vi "selectDevice.vi"(8 "error in (no error)":errorcluster, 9 "Custom Button 1":refnum<vi>, 10 "Custom Button 2":refnum<vi>, 11 "Daten in":T4={"Report.lvclass"=refnum, "Norm"="", "last State"=enum."Initialize", "Norm ID"=0, "EMTestCWS500N.lvclass"=refnum, "CEG4500.lvclass"=refnum, "Tektronix RSA5106A.lvclass"=refnum, "erfolgreich"=FALSE, "Device Enum"=enum."emTestCWS500N", "Test Enum"=enum."HF-Felder", "debug"=FALSE, "tab"=enum."Hauptmenü", "ESD Pistol.lvclass"=refnum, "SubPnl Refnum"=refnum, "TabCtl Refnum"=refnum, "ButtonsEinblenden?"=FALSE, "VKey"=enum."ASCII", "last Test"=refnum, "Class 4.lvclass"=refnum}) -> (0 "error out":errorcluster, 1 "DeviceInterface out":refnum<class "DeviceInterface.lvclass">, 2 "Burst.lvclass":refnum<class "TestInterface.lvclass">, 3 "Daten out":T4={"Report.lvclass"=refnum, "Norm"="", "last State"=enum."Initialize", "Norm ID"=0, "EMTestCWS500N.lvclass"=refnum, "CEG4500.lvclass"=refnum, "Tektronix RSA5106A.lvclass"=refnum, "erfolgreich"=FALSE, "Device Enum"=enum."emTestCWS500N", "Test Enum"=enum."HF-Felder", "debug"=FALSE, "tab"=enum."Hauptmenü", "ESD Pistol.lvclass"=refnum, "SubPnl Refnum"=refnum, "TabCtl Refnum"=refnum, "ButtonsEinblenden?"=FALSE, "VKey"=enum."ASCII", "last Test"=refnum, "Class 4.lvclass"=refnum}, 4 "Test Enum":T1, 5 "VISA resource name":refnum<visa-resource-name>, 6 "Device Enum":T2)   [LabVIEW 2013, in "EMV-Test.lvlib"]
uses:
  EMV-Test.lvlib
  classes/Devices/DeviceInterface/DeviceInterface.lvclass
  classes/Tests/Stoeraussendung/Stoeraussendung.lvclass
  classes/Tests/TestInterface/TestInterface.lvclass
  classes/Tests/Burst/Burst.lvclass
  classes/Tests/ESD/ESD.lvclass
  classes/Tests/Surge/Surge.lvclass
  classes/Tests/Spannungseinbruch/Spannungseinbruch.lvclass
  classes/Tests/HF-Felder/HF-Felder.lvclass
  Main/controls/TestStates.ctl
  classes/Tests/TestTest/TestTest.lvclass
  classes/Datastructure/Report/Report.lvclass
  Main/controls/State.ctl
  classes/Devices/emTestCWS500N/EMTestCWS500N.lvclass
  classes/Devices/CEG4500/CEG4500.lvclass
  classes/Devices/Tektronix RSA5106A/Tektronix RSA5106A.lvclass
  classes/Devices/DeviceInterface/Devices.ctl
  classes/Tests/TestInterface/Tests.ctl
  Main/controls/Data.ctl
  vis/Tabs.ctl
  vis/ESD Pistol.lvclass
  <vilib>/event_ctls.llb/eventvkey.ctl
  classes/Datastructure/Test/Test.lvclass
  classes/Devices/Class4/Class 4.lvclass
panel:
  out "Enum":T3
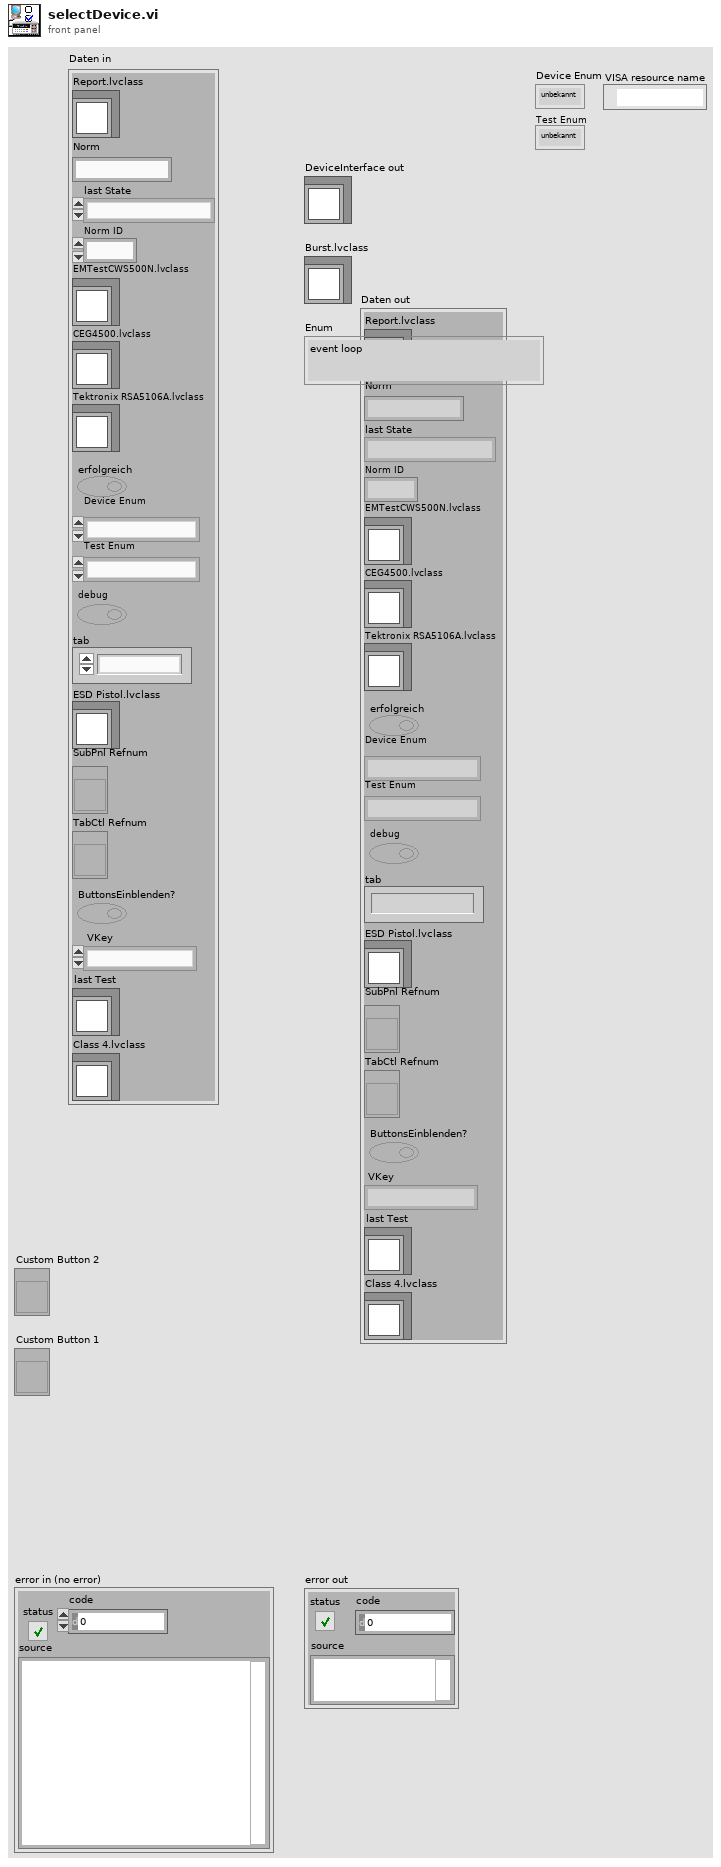
[diagram p1: front panel]
types:
  T1 = typedef "Tests.ctl" = enum16{"unbekannt", "Störaussendung", "Burst", "ESD", "Surge", "Spannungseinbruch", "HF-Felder"}
  T2 = typedef "Devices.ctl" = enum16{"unbekannt", "ESD Pistol", "Tektronix RSA5106A", "emTestCWS500N", "CEG-4500"}
  T3 = typedef "EMV-Test.lvlib/TestStates.ctl" = enum16{"event loop", "save Test", "Custom Action 1", "Custom Action 2", "pause", "vorgefertigter Test", "manueller Test", "respond to response", "error", "init", "start Test", "evaluate line", "wait for Response", "wait", "catch error", "close Connection", "end"}
  T4 = typedef "Data.ctl" = cluster{"Report.lvclass":refnum<class "Report.lvclass">, "Norm":string, "last State":T5, "Norm ID":i32, "EMTestCWS500N.lvclass":refnum<class "EMTestCWS500N.lvclass">, "CEG4500.lvclass":refnum<class "CEG4500.lvclass">, "Tektronix RSA5106A.lvclass":refnum<class "Tektronix RSA5106A.lvclass">, "erfolgreich":bool, "Device Enum":T2, "Test Enum":T1, "debug":bool, "tab":T6, "ESD Pistol.lvclass":refnum<class "ESD Pistol.lvclass">, "SubPnl Refnum":refnum<vi>, "TabCtl Refnum":refnum<vi>, "ButtonsEinblenden?":bool, "VKey":T7, "last Test":refnum<class "Test.lvclass">, "Class 4.lvclass":refnum<class "Class 4.lvclass">}
  T5 = typedef "State.ctl" = enum16{"create Pdf", "edit Report", "load Report", "save Report", "do Test", "CDN Kalibrierung", "enter Report Parameters", "new Test", "Protokoll", "read Tree", "update Tree", "Fehler", "Initialize", "Wait for Event", "Exit"}
  T6 = typedef "Tabs.ctl" = enum32{"Hauptmenü", "Prüfbericht", "Einstellungen"}
  T7 = typedef "eventvkey.ctl" = enum16{"ASCII", "Enter", "Return", "Shift", "Ctrl", "Alt", "Cmd", "Opt", "Caps", "NumLock", "Clear", "Break", "Up", "Down", "Left", "Right", "Insert", "Delete", "Home", "End", "PageUp", "PageDown", "Escape", "Help", "Pause", "ScrollLock", "F1", "F2", "F3", "F4", "F5", "F6", "F7", "F8", "F9", "F10", "F11", "F12", "F13", "F14", "F15", "F16", "F17", "F18", "F19", "F20", "F21", "F22", "F23", "F24", "Play", "VolumeUp", "VolumeDown", "Mute", "Two Byte Char"}
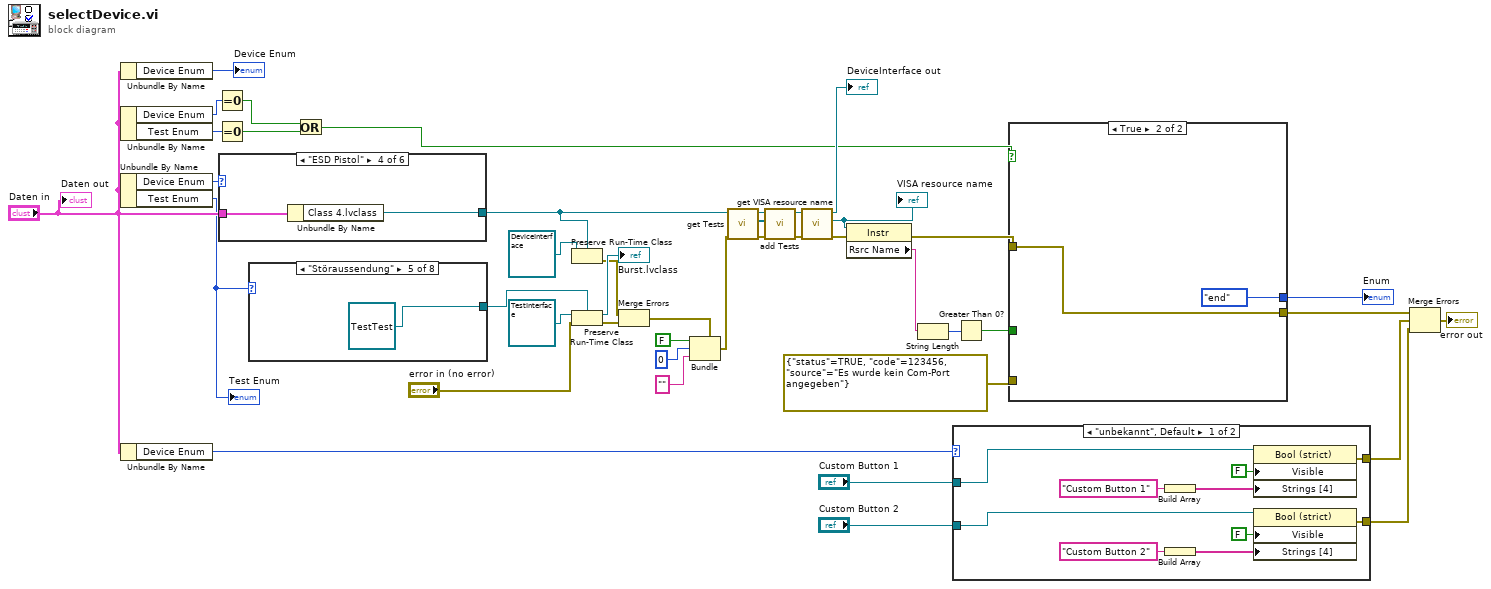
[diagram p0: block diagram]
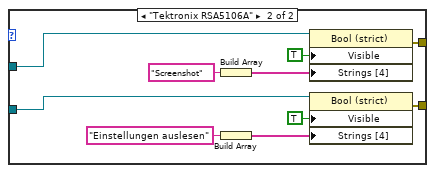
[diagram p2: hidden frame]
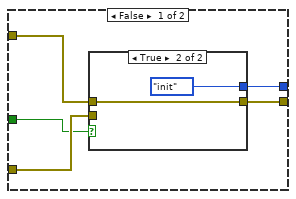
[diagram p3: hidden frame]
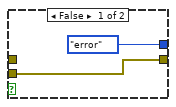
[diagram p4: hidden frame]
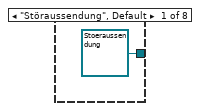
[diagram p5: hidden frame]
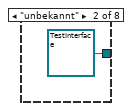
[diagram p6: hidden frame]
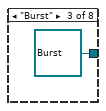
[diagram p7: hidden frame]
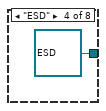
[diagram p8: hidden frame]
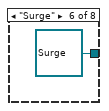
[diagram p9: hidden frame]
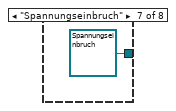
[diagram p10: hidden frame]
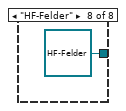
[diagram p11: hidden frame]
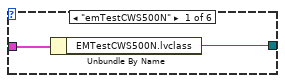
[diagram p12: hidden frame]
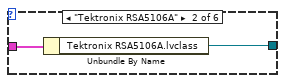
[diagram p13: hidden frame]
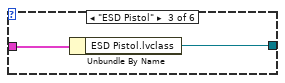
[diagram p14: hidden frame]
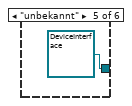
[diagram p15: hidden frame]
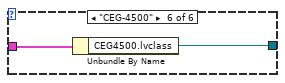
[diagram p16: hidden frame]
diagram:
  n1 = Unbundle By Name("Daten in") -> ("Device Enum"=→"Device Enum":T2)
  n2 = Unbundle By Name("Daten in") -> ("Device Enum"=w18:T2, "Test Enum"=w21:T1)
  n3 = Unbundle By Name("Daten in") -> ("Device Enum"=w28:T2, "Test Enum"=w29:T1)
  "Test Enum" <- w29
  n4 = Unbundle By Name("Daten in") -> ("Device Enum"=w33:T2)
  n5 = Equal To 0?(x=w18) -> (x = 0?=w19:bool)
  n6 = Equal To 0?(x=w21) -> (x = 0?=w20:bool)
  n7 = case shown="\"ESD Pistol\"" w28 {
    tunnel: [w44 w46 w48 w50 refnum<class "DeviceInterface.lvclass"> refnum ("Tektronix RSA5106A.lvclass") w53] -> w30
    tunnel: "Daten in" -> [w45 w47 w49 w51 _ w54]
    frame "emTestCWS500N" {
      n8 = Unbundle By Name(w45) -> ("EMTestCWS500N.lvclass"=w44:refnum<class "EMTestCWS500N.lvclass">)
    }
    frame "Tektronix RSA5106A" {
      n9 = Unbundle By Name(w47) -> ("Tektronix RSA5106A.lvclass"=w46:refnum<class "Tektronix RSA5106A.lvclass">)
    }
    frame "ESD Pistol" {
      n10 = Unbundle By Name(w49) -> ("ESD Pistol.lvclass"=w48:refnum<class "ESD Pistol.lvclass">)
    }
    frame "ESD Pistol" {
      n11 = Unbundle By Name(w51) -> ("Class 4.lvclass"=w50:refnum<class "Class 4.lvclass">)
    }
    frame "unbekannt" {
    }
    frame "CEG-4500" {
      n12 = Unbundle By Name(w54) -> ("CEG4500.lvclass"=w53:refnum<class "CEG4500.lvclass">)
    }
  }
  n13 = case shown="\"Störaussendung\"" w29 {
    tunnel: [refnum<class "Stoeraussendung.lvclass"> refnum ("Störaussendung.lvclass") refnum<class "TestInterface.lvclass"> refnum ("Burst.lvclass") refnum<class "Burst.lvclass"> refnum ("Burst.lvclass") refnum<class "ESD.lvclass"> refnum ("ESD.lvclass") refnum<class "TestTest.lvclass"> refnum ("TestTest.lvclass") refnum<class "Surge.lvclass"> refnum ("Surge.lvclass") refnum<class "Spannungseinbruch.lvclass"> refnum ("Spannungseinbruch.lvclass") refnum<class "HF-Felder.lvclass"> refnum ("HF-Felder.lvclass")] -> w6
    frame "Störaussendung", Default {
    }
    frame "unbekannt" {
    }
    frame "Burst" {
    }
    frame "ESD" {
    }
    frame "Störaussendung" {
    }
    frame "Surge" {
    }
    frame "Spannungseinbruch" {
    }
    frame "HF-Felder" {
    }
  }
  n14 = Or(x=w19, y=w20) -> (x .or. y?=w17:bool)
  n15 = Preserve Run-Time Class(object in=refnum<class "DeviceInterface.lvclass"> refnum ("DeviceInterface.lvclass"), 2:w30) -> (error out=w10:errorcluster)  [unwired: 1 in, 1 out]
  n16 = Preserve Run-Time Class(object in=refnum<class "TestInterface.lvclass"> refnum ("TestInterface.lvclass"), error in="error in (no error)", 2:w6) -> (object out=→"Burst.lvclass":refnum<class "TestInterface.lvclass">, error out=w7:errorcluster)
  n17 = Merge Errors(w10, w7) -> (w14:errorcluster)
  n18 = Bundle(cluster=w14, "status"=FALSE, "code"=0, "source"="") -> (w15:errorcluster)
  n19 = call-dynamic "get Tests.vi"("error in (no error)"=w15, "DeviceInterface (Eingang)"=w30) -> ("error out"=w23:errorcluster, "Tests"=w16:refnum<class "TestInterface.lvclass">[], "DeviceInterface (Ausgang)"=w24:refnum<class "DeviceInterface.lvclass">)  [unwired: 7 in]
  n20 = call-dynamic "add Tests.vi"("error in (no error)"=w23, "Tests"=w16, "DeviceInterface (Eingang)"=w24) -> ("error out"=w26:errorcluster, "DeviceInterface (Ausgang)"=w25:refnum<class "DeviceInterface.lvclass">)  [unwired: 7 in]
  n21 = call-dynamic "get VISA resource name.vi"("error in (no error)"=w26, "DeviceInterface (Eingang)"=w25) -> ("error out"=w37:errorcluster, "VISA resource name"=w36:refnum<visa-resource-name>, "DeviceInterface (Ausgang)"=→"DeviceInterface out":refnum<class "DeviceInterface.lvclass">)  [unwired: 7 in]
  "VISA resource name" <- w36
  n22 = property class="Instr"(reference=w36, error in=w37) -> (error out=w38:errorcluster, "Rsrc Name"=w41:string)  [unwired: 1 out]
  n23 = String Length(string=w41) -> (length=w39:i32)
  n24 = case shown="\"unbekannt\", Default" w33 {
    tunnel: [w71 w81] -> w32
    tunnel: [w65 w75] -> w43
    tunnel: "Custom Button 1" -> [w64 w73]
    tunnel: "Custom Button 2" -> [w63 w74]
    frame "unbekannt", Default {
      n25 = Build Array("Custom Button 1" ("Label.Text")) -> (w69:string[])
      n26 = Build Array("Custom Button 2" ("Label.Text")) -> (w68:string[])
      n27 = property class="Bool (strict)"(reference=w64, "Visible"=FALSE, "Strings [4]"=w69) -> (error out=w71:errorcluster)  [unwired: 1 in, 1 out]
      n28 = property class="Bool (strict)"(reference=w63, "Visible"=FALSE, "Strings [4]"=w68) -> (error out=w65:errorcluster)  [unwired: 1 in, 1 out]
    }
    frame "Tektronix RSA5106A" {
      n29 = Build Array("Screenshot" ("Label.Text")) -> (w79:string[])
      n30 = Build Array("Einstellungen auslesen" ("Label.Text")) -> (w78:string[])
      n31 = property class="Bool (strict)"(reference=w73, "Visible"=TRUE, "Strings [4]"=w79) -> (error out=w81:errorcluster)  [unwired: 1 in, 1 out]
      n32 = property class="Bool (strict)"(reference=w74, "Visible"=TRUE, "Strings [4]"=w78) -> (error out=w75:errorcluster)  [unwired: 1 in, 1 out]
    }
  }
  n33 = Greater Than 0?(x=w39) -> (x > 0?=w40:bool)
  n34 = case shown="True" w17 {
    tunnel: [w87 TestStates."end" ("Enum")] -> w22
    tunnel: [w86 w92] -> w35
    tunnel: errorcluster {"status"=TRUE, "code"=123456, "source"="Es wurde kein Com-Port angegeben"} ("error out") -> [w85 _]
    tunnel: w38 -> [w84 w92]
    tunnel: w40 -> [w83 _]
    frame False {
      n35 = case shown="True" w83 {
        tunnel: [TestStates."error" ("Enum") TestStates."init" ("Enum")] -> w87
        tunnel: [w88 w90] -> w86
        tunnel: w85 -> [w88 _]
        tunnel: w84 -> [_ w90]
        frame False {
        }
        frame True {
        }
      }
    }
    frame True {
    }
  }
  "Enum" <- w22
  n36 = Merge Errors(w35, w32, w43) -> (→"error out":errorcluster)
  "Daten out" <- "Daten in"
